vi "3-Rotina de aquisição dos dados de calibração.vi"() -> ()   [LabVIEW 2011]
uses:
  <vilib>/Analysis/NI_AALPro.lvlib
  <vilib>/Analysis/polynomials.llb/1D Polynomial Evaluation (DBL).vi
  <vilib>/Instr/_visa.llb/VISA Configure Serial Port (Instr).vi
panel:
  in  "Parâmetros de Calibração":path
  out "calibracao":dbl[](array[numeric])
  out "esquerdo":dbl
  out "direito":dbl
  in  "OK Button":bool
  in  "Parar Programa":bool
  out "Waveform Graph":dbl[](graph)
  out "submatrix":dbl[][](array[numeric])
  out "String Concatenada":string
  in  "Parar Aquisição do Sinal":bool
  out "Sinal":dbl[](graph)
  out "Tempo de Espera para cada iteração:":dbl caption="Elapsed Time (s)"
  out "Delay Sofrido em cada iteração":u32
  in  "Delay sofrido em cada iteração:":u32
  in  "VISA Resource: Name:":refnum<visa-resource-name>
  in  "Baud Rate:":u32=9600
  # "COMO USAR ESTE PROGRAMA:\n1º   Clique no ícone da pasta para\n       abrir os parâmetros de calibração.\n2º   Insira em VISA resorce Name o \n       valor da porta USB onde está \n       conectado o cabo do receptor.\n3º   Insira o valor Baud Rate com o \n       qual o arduino está programado.\n4º   Insira o valor de tempo de espera\n       sofrido por cada iteração do \n       programa\n5º   Coloque  o carregamento e espere\n       a haste estabilizar a oscilação\n6º   Execute o programa\n7º   Depois de um instante, pare a \n       aquisição dos  dados, clique em \n       Parar Aquisição\n8º   Selecione a região de interesse dos\n      dados que deseje salvar\n9º   Clicar em gravar e escreva o nome\n      do arquivo. Lembre-se de inserir\n      a extensão \".txt\"\n10º Finalizar o programa clicando em \n       Parar Programa\n11º Se precisar inserir  um novo \n      carregamente, repetir a sequência\n       a partir do 5º passo."
  # "ROTINA DE AQUISI敲O DOS DADOS DE CALIBRA敲O"
  # "SINAL AQUISITADO EM TEMPO REAL"
  # "Abrir Parâmetros de Regressão:"
  # "ms"
  # "ms"
  # "ms"
  # "SINAL A SER GRAVADO PARA PROCESSAMENTO"
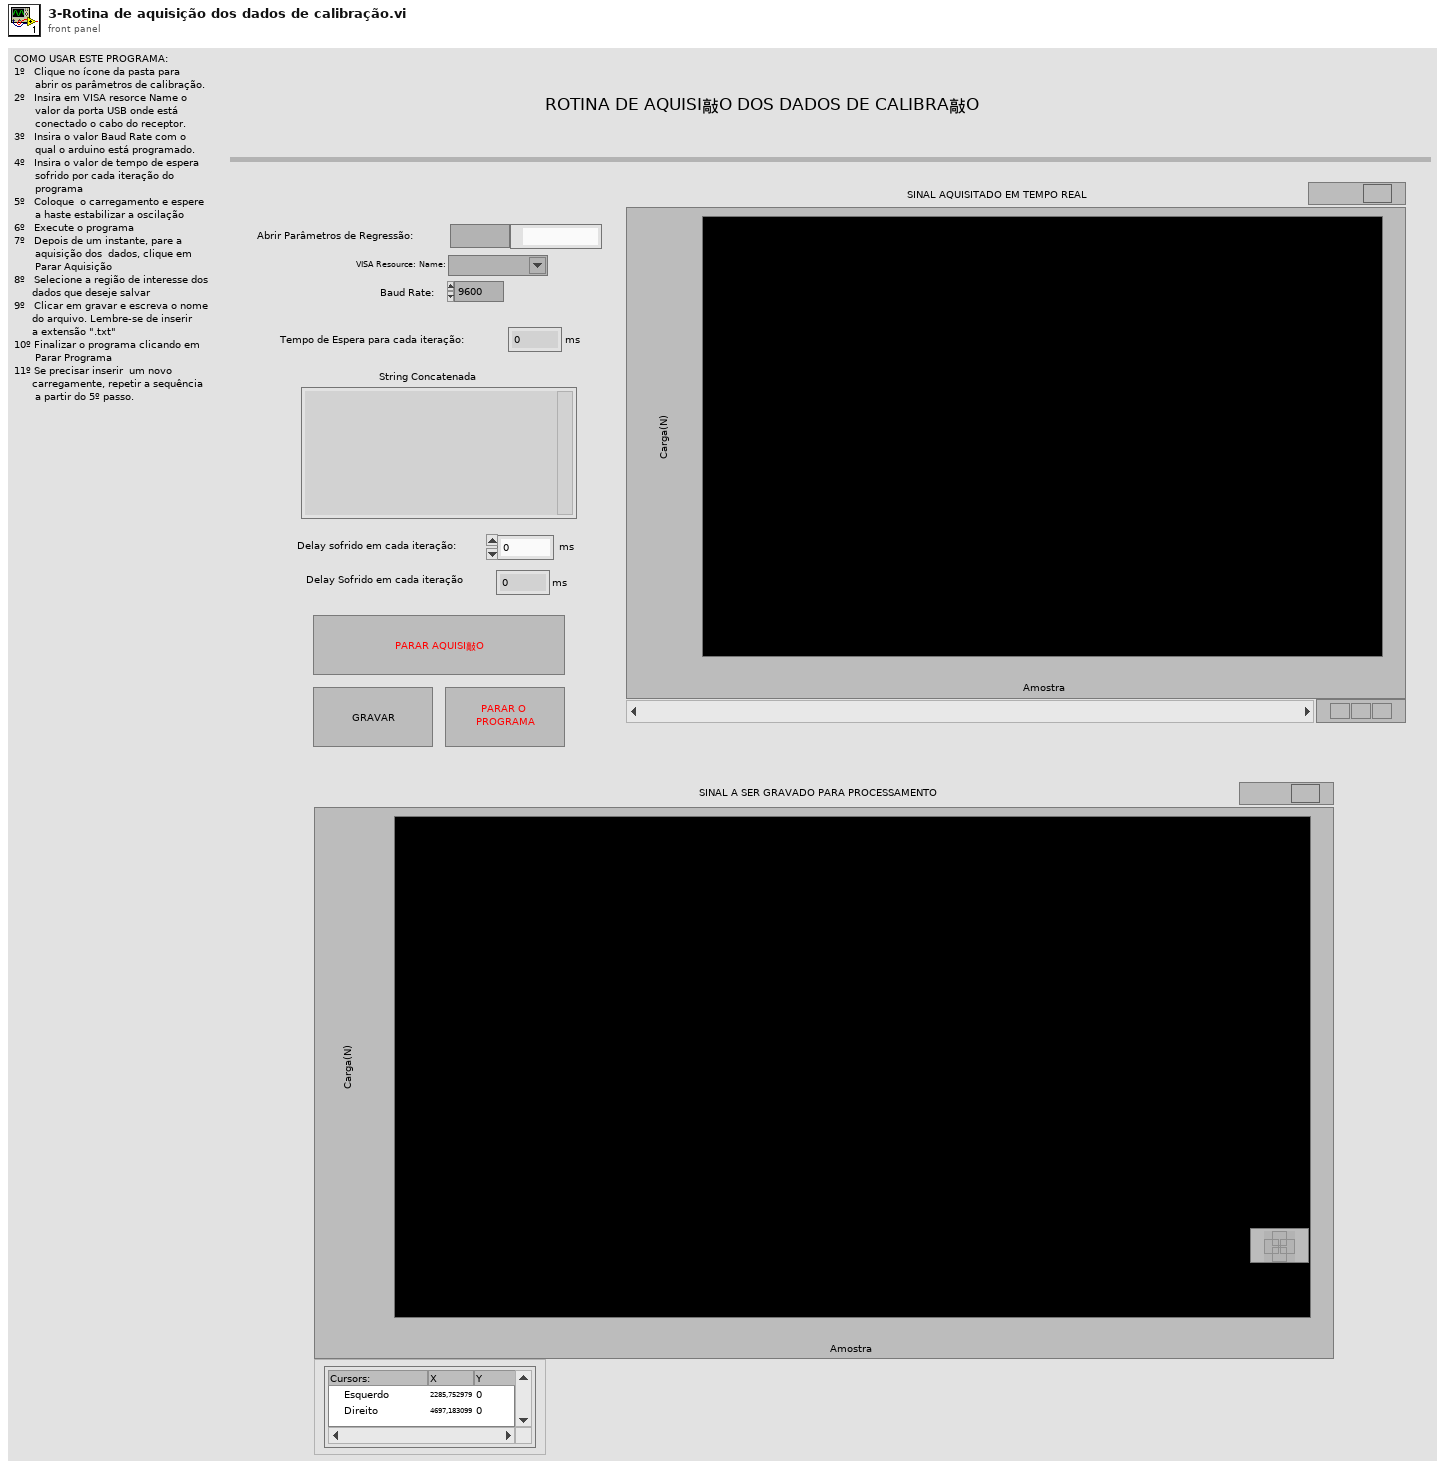
[diagram p1: front panel]
types:
  T1 = typedef "NI_Matrix.lvlib/RealMatrix.ctl" = dbl[][]
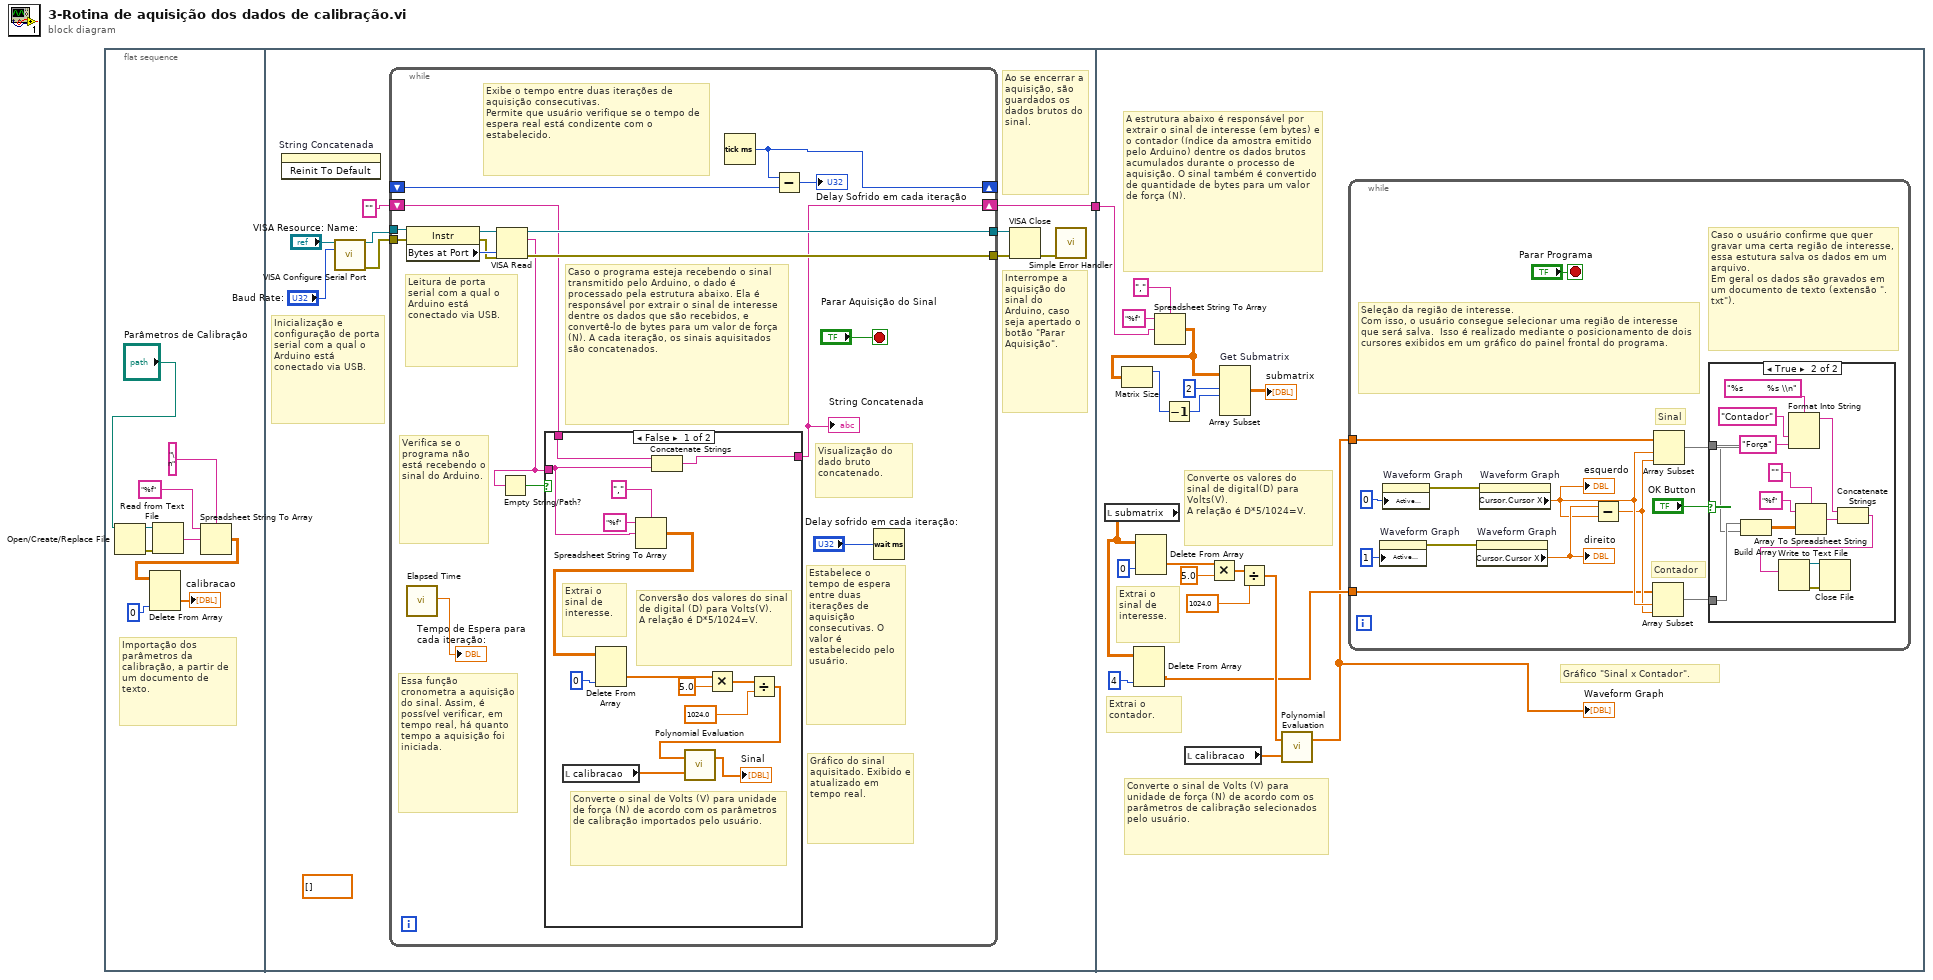
[diagram p0: block diagram]
diagram:
  n1 = flat-sequence {
    tunnel: [w11] -> w1
    tunnel: w1 -> [w56]
    frame #0 {
      # "Importação dos parâmetros da calibração, a partir de um documento de texto."
      n2 = Open/Create/Replace File(file path (use dialog)="Parâmetros de Calibração") -> (refnum out=w4:refnum<file>, error out=w5:errorcluster)  [unwired: 5 in, 1 out]
      n3 = Read from Text File(file (use dialog)=w4, error in=w5) -> (text=w3:string)  [unwired: 2 in, 3 out]
      n4 = Spreadsheet String To Array(delimiter (Tab)="\n", format string="%f", spreadsheet string=w3) -> (array=w9:dbl[][])  [unwired: 1 in]
      n5 = Delete From Array(array=w9, index (col)=0 ("disabled index (col)")) -> (deleted portion=→"calibracao":dbl[])  [unwired: 2 in, 1 out]
    }
    frame #1 {
      (unwired) dbl[] [] ("array")
      # "Interrompe a aquisição do sinal do Arduino, caso seja apertado o botão \"Parar Aquisição\"."
      # "Ao se encerrar a aquisição, são guardados os dados brutos do sinal."
      # "Inicialização e configuração de porta serial com a qual o Arduino está conectado via USB."
      n6 = invoke on="String Concatenada" class="Str" method="Reinit To Default"() -> ()  [unwired: 3 in, 3 out]
      n7 = call-poly "VISA Configure Serial Port"("VISA resource name"="VISA Resource: Name:", "baud rate (9600)"="Baud Rate:") -> ("VISA resource name out"=w19:refnum<visa-resource-name>, "error out"=w18:errorcluster)  [unwired: 12 in]
      n8 = while {
        tunnel: w19 -> [w36]
        tunnel: w18 -> [w35]
        tunnel: [w32] -> w14
        tunnel: [w31] -> w13
        shift-right: [w21] -> w11
        shift-left: "" -> [w22]
        shift-right: [w20] -> _
        shift-left: _ -> [w27]
        stop <- "Parar Aquisição do Sinal" stop-if-true
        # "Visualização do dado bruto concatenado."
        # "Estabelece o tempo de espera entre duas iterações de aquisição consecutivas. O valor é estabelecido pelo usuário."
        # "Gráfico do sinal aquisitado. Exibido e atualizado em tempo real."
        # "Leitura de porta serial com a qual o Arduino está conectado via USB."
        # "Exibe o tempo entre duas iterações de aquisição consecutivas. \nPermite que usuário verifique se o tempo de espera real está condizente com o estabelecido."
        # "Caso o programa esteja recebendo o sinal transmitido pelo Arduino, o dado é processado pela estrutura abaixo. Ela é responsável por extrair o sinal de interesse dentre os dados que são recebidos, e convertê-lo de bytes para um valor de força (N). A cada iteração, os sinais aquisitados são concatenados."
        # "Verifica se o programa não está recebendo o sinal do Arduino."
        # "Essa função cronometra a aquisição do sinal. Assim, é possível verificar, em tempo real, há quanto tempo a aquisição foi iniciada."
        n9 = property class="Instr"(reference=w36, error in=w35) -> (reference out=w34:refnum<visa-resource-name>, error out=w29:errorcluster, "Bytes at Port"=w33:u32)
        n10 = call "Elapsed Time"() -> ("Elapsed Time (s)"=→"Tempo de Espera para cada iteração:":dbl)  [unwired: 12 in, 7 out]
        n11 = VISA Read(VISA resource name=w34, byte count=w33, error in (no error)=w29) -> (VISA resource name out=w32:refnum<visa-resource-name>, read buffer=w24:string, error out=w31:errorcluster)  [unwired: 1 out]
        n12 = Empty String/Path?(string/path=w24) -> (empty?=w23:bool)
        n13 = case shown="False" w23 {
          tunnel: w24 -> [w38 _]
          tunnel: w22 -> [w41 w51]
          tunnel: [w40 w51] -> w21
          frame False {
            # "Converte o sinal de Volts (V) para unidade de força (N) de acordo com os parâmetros de calibração importados pelo usuário."
            # "Conversão dos valores do sinal de digital (D) para Volts(V).\nA relação é D*5/1024=V."
            # "Extrai o sinal de interesse."
            n14 = local read "calibracao"() -> (w42:dbl[])
            n15 = Spreadsheet String To Array(delimiter (Tab)=",", format string="%f", spreadsheet string=w38) -> (array=w44:dbl[][])  [unwired: 1 in]
            n16 = Delete From Array(array=w44, index (col)=0 ("disabled index (col)")) -> (deleted portion=w45:dbl[])  [unwired: 2 in, 1 out]
            n17 = Concatenate Strings(w41, w38) -> (w40:string)
            n18 = Multiply(x=w45, y=5.0) -> (x*y=w47:dbl[])
            n19 = Divide(x=w47, y=1024.0) -> (x/y=w43:dbl[])
            n20 = call-poly <vilib>:"Polynomial Evaluation.vi"("P(x)"=w42, "A"=w43) -> ("P(A)"=→"Sinal":dbl[])  [unwired: 1 out]
          }
          frame True {
          }
        }
        "String Concatenada" <- w21
        n21 = Tick Count (ms)() -> (millisecond timer value=w20:u32)
        n22 = Subtract(x=w20, y=w27) -> (x-y=→"Delay Sofrido em cada iteração":u32)
        n23 = Wait (ms)(milliseconds to wait="Delay sofrido em cada iteração:") -> ()  [unwired: 1 out]
      }
      n24 = VISA Close(VISA resource name=w14, error in (no error)=w13) -> (error out=w12:errorcluster)
      n25 = call <vilib>:"Simple Error Handler.vi"("error in (no error)"=w12) -> ()  [unwired: 1 in, 8 out]
    }
    frame #2 {
      # "Gráfico \"Sinal x Contador\"."
      # "Converte o sinal de Volts (V) para unidade de força (N) de acordo com os parâmetros de calibração selecionados pelo usuário."
      # "Converte os valores do\nsinal de digital(D) para Volts(V).\nA relação é D*5/1024=V."
      # "A estrutura abaixo é responsável por extrair o sinal de interesse (em bytes) e o contador (índice da amostra emitido pelo Arduino) dentre os dados brutos acumulados durante o processo de aquisição. O sinal também é convertido de quantidade de bytes para um valor de força (N)."
      # "Extrai o contador."
      # "Extrai o sinal de interesse."
      n26 = local read "submatrix"() -> (w61:dbl[][])
      n27 = Delete From Array(array=w61, index (col)=4 ("disabled index (col)")) -> (deleted portion=w53:dbl[])  [unwired: 2 in, 1 out]
      n28 = Delete From Array(array=w61, index (col)=0 ("disabled index (col)")) -> (deleted portion=w57:dbl[])  [unwired: 2 in, 1 out]
      n29 = Spreadsheet String To Array(delimiter (Tab)=",", format string="%f", spreadsheet string=w56) -> (array=w68:dbl[][])  [unwired: 1 in]
      n30 = Matrix Size(0:w68) -> (1:w66:i32)  [unwired: 1 out]
      n31 = Decrement(x=w66) -> (x-1=w65:i32)
      n32 = local read "calibracao"() -> (w54:dbl[])
      n33 = Multiply(x=w57, y=5.0) -> (x*y=w59:dbl[])
      n34 = Array Subset "Get Submatrix"(array=w68, index (row)=2, length (row)=w65) -> (→"submatrix":dbl[][])  [unwired: 2 in]
      n35 = Divide(x=w59, y=1024.0) -> (x/y=w55:dbl[])
      n36 = call-poly <vilib>:"Polynomial Evaluation.vi"("P(x)"=w54, "A"=w55) -> ("P(A)"=w52:dbl[])  [unwired: 1 out]
      "Waveform Graph" <- w52
      n37 = while {
        tunnel: w53 -> [w73]
        tunnel: w52 -> [w71]
        stop <- "Parar Programa" stop-if-true
        # "Caso o usuário confirme que quer gravar uma certa região de interesse, essa estutura salva os dados em um arquivo.\nEm geral os dados são gravados em um documento de texto (extensão \".txt\")."
        # "Seleção da região de interesse. \nCom isso, o usuário consegue selecionar uma região de interesse que será salva.  Isso é realizado mediante o posicionamento de dois cursores exibidos em um gráfico do painel frontal do programa."
        # "Contador"
        # "Sinal"
        n38 = property on="Waveform Graph" class="WFGraph (strict)"("Active Cursor"=u32 1) -> (error out=w81:errorcluster)  [unwired: 2 in, 1 out]
        n39 = property on="Waveform Graph" class="WFGraph (strict)"("Active Cursor"=u32 0) -> (error out=w83:errorcluster)  [unwired: 2 in, 1 out]
        n40 = property on="Waveform Graph" class="WFGraph (strict)"(error in=w81) -> ("Cursor.Cursor X"=w79:dbl)  [unwired: 1 in, 2 out]
        "direito" <- w79
        n41 = property on="Waveform Graph" class="WFGraph (strict)"(error in=w83) -> ("Cursor.Cursor X"=w75:dbl)  [unwired: 1 in, 2 out]
        "esquerdo" <- w75
        n42 = Subtract(x=w79, y=w75) -> (x-y=w74:dbl)
        n43 = Array Subset(array=w73, index=w75, length=w74) -> (w72:dbl[])
        n44 = Array Subset(array=w71, index=w75, length=w74) -> (w77:dbl[])
        n45 = case shown="True" "OK Button" {
          tunnel: w77 -> [_ w84]
          tunnel: w72 -> [_ w85]
          frame False {
          }
          frame True {
            n46 = Build Array(w85, w84) -> (w89:T1)
            n47 = Format Into String(format string="%s        %s \\n", "Contador" ("input 1"), "Força" ("input 2")) -> (resulting string=w90:string)  [unwired: 2 in, 1 out]
            n48 = Array To Spreadsheet String(delimiter (Tab)="", array=w89, 3:"%f" ("format string")) -> (spreadsheet string=w91:string)
            n49 = Concatenate Strings(w90, w91) -> (w86:string)
            n50 = Write to Text File(text=w86) -> (refnum out=w88:refnum<file>, error out=w87:errorcluster)  [unwired: 3 in, 1 out]
            n51 = Close File(refnum=w88, error in=w87) -> ()  [unwired: 2 out]
          }
        }
      }
    }
  }
